vi "set offset tuning.vi"(8 "error in (no error)":errorcluster, 10 "Offset Tuning":bool, 11 "DeviceRefnum":u64) -> (0 "error out":errorcluster, 2 "function return":i32, 3 "DeviceRefnum Out":u64)   [LabVIEW 2015, in "rtlsdr.lvlib"]
doc: "Enable or disable offset tuning for zero-IF tuners, which allows to avoid problems caused by the DC offset of the ADCs and 1/f noise."
uses:
  rtlsdr.lvlib
  rtlsdr/rtlsdr.dll
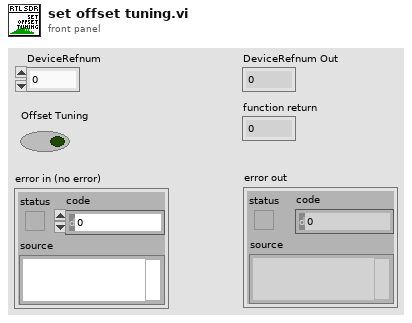
[diagram p1: front panel]
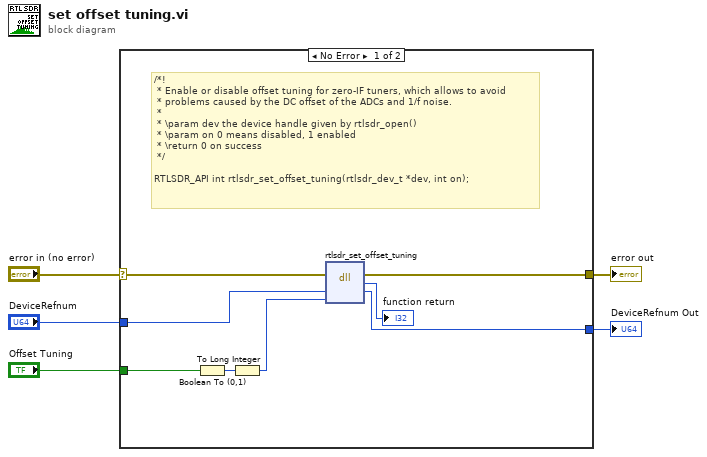
[diagram p0: block diagram]
diagram:
  n1 = case shown="No Error" "error in (no error)" {
    selector: "error in (no error)" -> [w6 w15]
    tunnel: [w12 w15] -> w5
    tunnel: "DeviceRefnum" -> [w11 w14]
    tunnel: [w10 w14] -> w3
    tunnel: "Offset Tuning" -> [w8 _]
    frame No Error {
      # "/*!\n * Enable or disable offset tuning for zero-IF tuners, which allows to avoid\n * problems caused by the DC offset of the ADCs and 1/f noise.\n *\n * \\param dev the device handle given by rtlsdr_open()\n * \\param on 0 means disabled, 1 enabled\n * \\return 0 on success\n */\n\nRTLSDR_API int rtlsdr_set_offset_tuning(rtlsdr_dev_t *dev, int on);"
      n2 = Boolean To (0,1)(Boolean=w8) -> (0, 1=w9:i16)
      n3 = To Long Integer(number=w9) -> (32bit integer=w7:i32)
      n4 = dll-call lib="C:/Users/TheDoctor/Documents/Projects/Labview Libraries/rtlsdr/rtlsdr.*" fn="rtlsdr_set_offset_tuning"(error in=w6, "DeviceRefnum"=w11, "Offset Tuning"=w7) -> (error out=w12:errorcluster, "return type"=→"function return":i32, "DeviceRefnum"=w10:u64)  [unwired: 3 in, 1 out]
    }
    frame Error {
    }
  }
  "error out" <- w5
  "DeviceRefnum Out" <- w3
